vi "Pipelined Processing (Optimized Performance).vi"() -> ()   [LabVIEW 2023]
doc: "The Pipelined Processing (Optimized Performance) example shows how to use feedback nodes to allow different processing functions to operate on different images in the same cycle. This example uses a ring acquisition which is optimized for performance, but has some restrictions on the camera's image format and size. Use the Pipelined Processing VI if your camera settings do not work with a ring acquisition.\n\nIn this example, image processing is simulated by a time delay that can be adjusted while the VI is running. When processing is complete, <B>IMAQdx Release Image</B> must be called in order to free space in the ring buffer."
uses:
  <vilib>/vision/driver/IMAQdx.llb/IMAQdx Acquisition Mode.ctl
  <vilib>/vision/driver/IMAQdx.llb/IMAQdx Buffer Number Mode.ctl
  <vilib>/vision/Image Controls.llb/IMAQ Image.ctl
  <vilib>/vision/driver/NI_Vision_Acquisition_Software.lvlib
panel:
  in  "Processing Delay (ms)":dbl=5.0
  out "Image":T1(plugin-control)
  out "Acquired Frame Rate":dbl
  out "Processing Frame Rate":dbl
  in  "Enable Pipelined Processing":bool
  out "Lost Buffer Count":u32
  in  "Number of Images":i32=30
  in  "Camera Name":refnum<k21> caption="IMAQdx Session"
  in  "Stop":bool
  # "Overview: Demonstrates how to process an image using a pipelined approach to improve performance so multiple operations can happen on the same iteration of the loop.\nRequirements: Vision Acquisition Software\nInstructions:\n1. Select the Camera Name\n2. Run the VI and increase the Processing Delay until the Processing Frame Rate is less than the Acquired Frame Rate\n3. Stop the VI and turn on the Enabled Pipelined Processing and repeat step 2 to compare the maximum Processing Delay before falling behind"
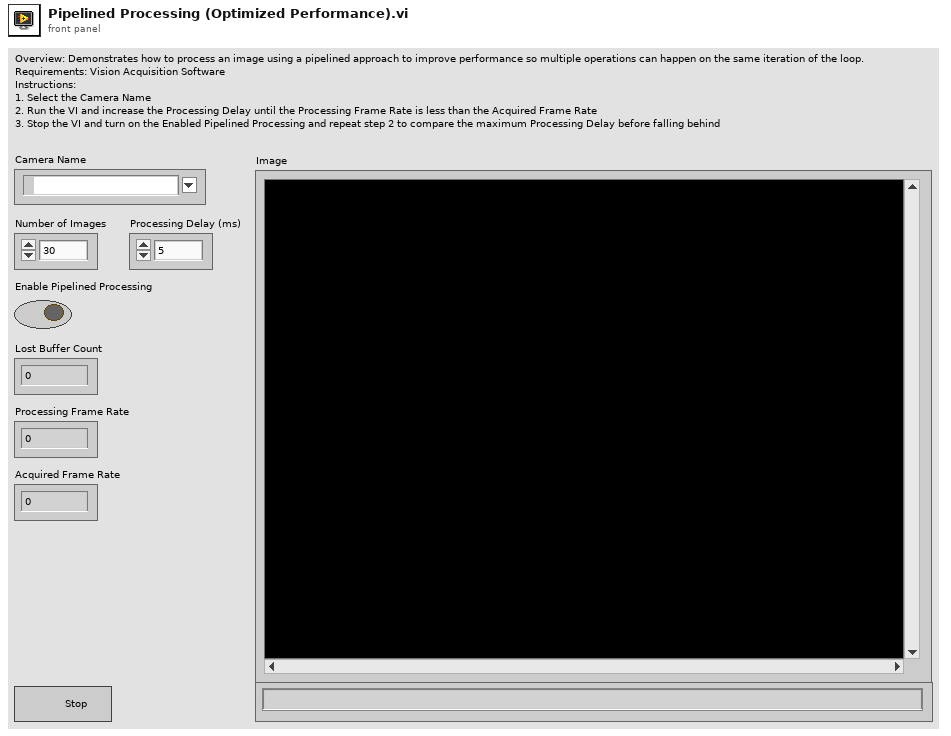
[diagram p1: front panel]
types:
  T1 = typedef "IMAQ Image.ctl" = refnum<image>
  T2 = typedef "NI_Vision_Acquisition_Software.lvlib/IMAQdx Acquisition Mode.ctl" = enum32{"One Shot", "Continuous"}
  T3 = typedef "IMAQdx.ctl" = refnum<k21>
  T4 = typedef "NI_Vision_Acquisition_Software.lvlib/IMAQdx Buffer Number Mode.ctl" = enum32{"Next", "Last", "Buffer Number", "Every", "Last New"}
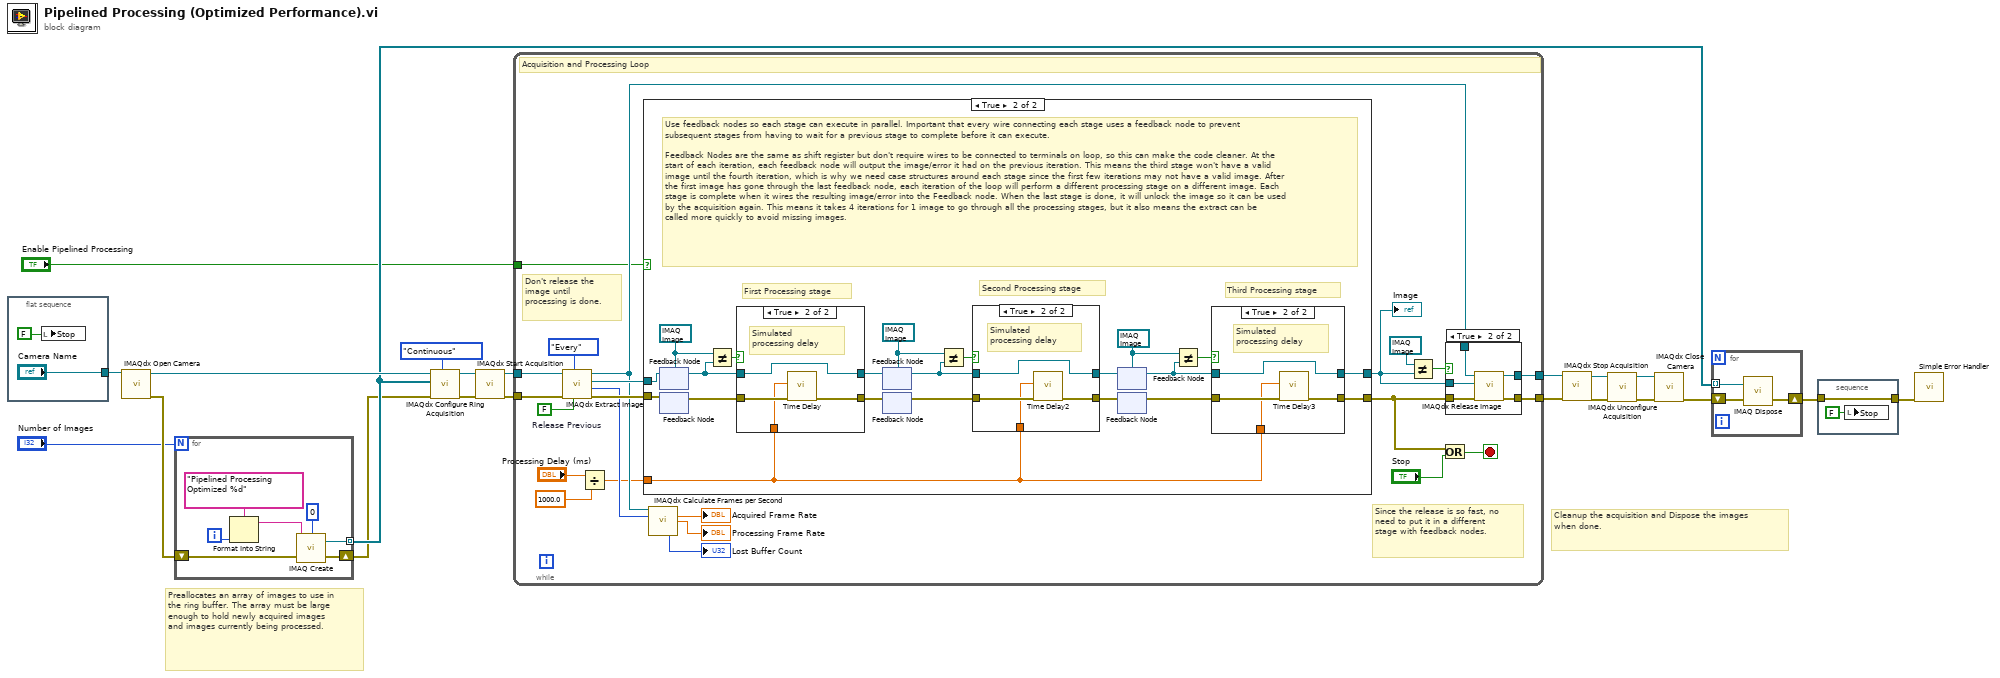
[diagram p0: block diagram]
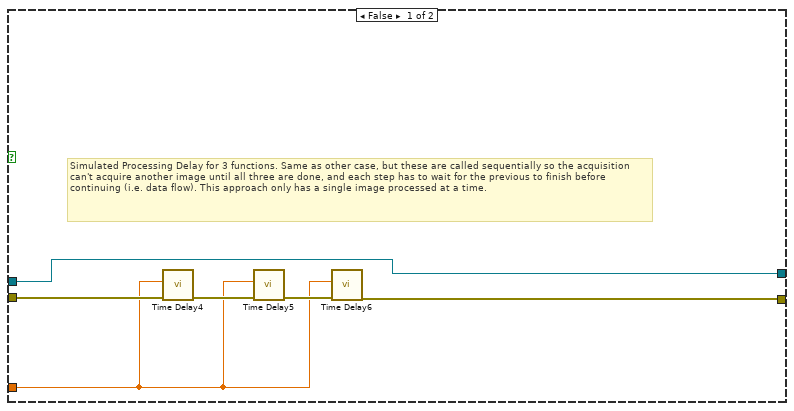
[diagram p2: hidden frame]
diagram:
  # "Cleanup the acquisition and Dispose the images when done."
  # "Preallocates an array of images to use in the ring buffer. The array must be large enough to hold newly acquired images and images currently being processed."
  n1 = flat-sequence {
    tunnel: ["Camera Name"] -> w20
    frame #0 {
      n2 = local write "Stop"(FALSE ("Stop")) -> ()
    }
  }
  n3 = call <vilib>:"IMAQdx Open Camera.vi"("Session In"=w20) -> ("error out"=w13:errorcluster, "Session Out"=w12:T3)  [unwired: 2 in, 7 out]
  n4 = for {
    N: "Number of Images" -> [_]
    tunnel: [w29] -> w9 mode=indexing
    shift-right: [w28] -> w4
    shift-left: w13 -> [w30]
    i -> [w27]
    n5 = Format Into String(format string="Pipelined Processing Optimized %d" ("Image Name"), w27) -> (resulting string=w26:string)  [unwired: 2 in, 1 out]
    n6 = call "IMAQ Create"("Border Size"=0, "Image Name"=w26, "error in (no error)"=w30) -> ("New Image"=w29:T1, "error out"=w28:errorcluster)  [unwired: 1 in, 1 out]
  }
  n7 = call <vilib>:"IMAQdx Configure Ring Acquisition.vi"("Mode"=IMAQdx_Acquisition_Mode."Continuous" ("Continuous?"), "error in"=w4, "Images"=w9, "Session In"=w12) -> ("error out"=w14:errorcluster, "Session Out"=w15:T3)  [unwired: 5 in, 1 out]
  n8 = call <vilib>:"IMAQdx Start Acquisition.vi"("error in"=w14, "Session In"=w15) -> ("error out"=w21:errorcluster, "Session Out"=w7:T3)  [unwired: 8 out]
  n9 = while {
    tunnel: w21 -> [w53]
    tunnel: w7 -> [w49]
    tunnel: [w41] -> w8
    tunnel: [w42] -> w1
    tunnel: "Enable Pipelined Processing" -> [w35]
    stop <- w36 stop-if-true
    w50 = FALSE  # Release Previous
    # "Since the release is so fast, no need to put it in a different stage with feedback nodes."
    # "Don't release the image until processing is done."
    # "Acquisition and Processing Loop"
    n10 = call <vilib>:"IMAQdx Extract Image.vi"("Release Previous (true)"=w50, "Buffer Number Mode (Next)"=IMAQdx_Buffer_Number_Mode."Every" ("Buffer Number Mode"), "error in"=w53, "Session In"=w49) -> ("error out"=w47:errorcluster, "Buffer Number Out"=w38:u32, "Image Out"=w46:T1, "Session Out"=w40:T3)  [unwired: 4 in]
    n11 = Divide(x="Processing Delay (ms)", y=1000.0) -> (x/y=w32:dbl)
    n12 = case shown="True" w35 {
      tunnel: w47 -> [w59 w80]
      tunnel: w46 -> [w55 w79]
      tunnel: [w56 w78] -> w43
      tunnel: [w55 w64] -> w31
      tunnel: w32 -> [w54 w60]
      frame False {
        # "Simulated Processing Delay for 3 functions. Same as other case, but these are called sequentially so the acquisition can't acquire another image until all three are done, and each step has to wait for the previous to finish before continuing (i.e. data flow). This approach only has a single image processed at a time."
        n13 = call "Time Delay4"("error in (no error)"=w59, "Delay Time (s)"=w54) -> ("error out"=w58:errorcluster)  [unwired: 9 in]
        n14 = call "Time Delay5"("error in (no error)"=w58, "Delay Time (s)"=w54) -> ("error out"=w57:errorcluster)  [unwired: 9 in]
        n15 = call "Time Delay6"("error in (no error)"=w57, "Delay Time (s)"=w54) -> ("error out"=w56:errorcluster)  [unwired: 9 in]
      }
      frame True {
        w61 = T1 refnum ("Image Out")
        w62 = T1 refnum ("Image Out")
        w63 = T1 refnum ("Image Out")
        # "Use feedback nodes so each stage can execute in parallel. Important that every wire connecting each stage uses a feedback node to prevent subsequent stages from having to wait for a previous stage to complete before it can execute.\n\nFeedback Nodes are the same as shift register but don't require wires to be connected to terminals on loop, so this can make the code cleaner. At the start of each iteration, each feedback node will output the image/error it had on the previous iteration. This means the third stage won't have a valid image until the fourth iteration, which is why we need case structures around each stage since the first few iterations may not have a valid image. After the first image has gone through the last feedback node, each iteration of the loop will perform a different processing stage on a different image. Each stage is complete when it wires the resulting image/error into the Feedback node. When the last stage is done, it will unlock the image so it can be used by the acquisition again. This means it takes 4 iterations for 1 image to go through all the processing stages, but it also means the extract can be called more quickly to avoid missing images."
        # "Third Processing stage"
        # "Second Processing stage"
        # "First Processing stage"
        n16 = feedback #1(w63) -> (w66:T1)
        n17 = feedback-in #1(w79) -> ()
        n18 = feedback #2() -> (w77:errorcluster)  [unwired: 1 in]
        n19 = feedback-in #2(w80) -> ()
        n20 = Not Equal?(x=w63, y=w66) -> (x != y?=w65:bool)
        n21 = case shown="True" w65 {
          tunnel: w77 -> [w93 w98]
          tunnel: w66 -> [w94 w95]
          tunnel: [w94 w95] -> w76
          tunnel: [w93 w97] -> w75
          tunnel: w60 -> [_ w96]
          frame False {
            # "No image to process"
          }
          frame True {
            # "Simulated processing delay"
            n22 = call "Time Delay"("error in (no error)"=w98, "Delay Time (s)"=w96) -> ("error out"=w97:errorcluster)  [unwired: 9 in]
          }
        }
        n23 = feedback #3(w62) -> (w73:T1)
        n24 = feedback-in #3(w76) -> ()
        n25 = feedback #4() -> (w72:errorcluster)  [unwired: 1 in]
        n26 = feedback-in #4(w75) -> ()
        n27 = Not Equal?(x=w62, y=w73) -> (x != y?=w74:bool)
        n28 = case shown="True" w74 {
          tunnel: w72 -> [w87 w92]
          tunnel: w73 -> [w88 w89]
          tunnel: [w88 w89] -> w71
          tunnel: [w87 w91] -> w70
          tunnel: w60 -> [_ w90]
          frame False {
            # "No image to process"
          }
          frame True {
            # "Simulated processing delay"
            n29 = call "Time Delay2"("error in (no error)"=w92, "Delay Time (s)"=w90) -> ("error out"=w91:errorcluster)  [unwired: 9 in]
          }
        }
        n30 = feedback #5(w61) -> (w69:T1)
        n31 = feedback-in #5(w71) -> ()
        n32 = feedback #6() -> (w68:errorcluster)  [unwired: 1 in]
        n33 = feedback-in #6(w70) -> ()
        n34 = Not Equal?(x=w61, y=w69) -> (x != y?=w67:bool)
        n35 = case shown="True" w67 {
          tunnel: w68 -> [w81 w86]
          tunnel: w69 -> [w82 w83]
          tunnel: [w82 w83] -> w64
          tunnel: [w81 w85] -> w78
          tunnel: w60 -> [_ w84]
          frame False {
            # "No image to process"
          }
          frame True {
            # "Simulated processing delay"
            n36 = call "Time Delay3"("error in (no error)"=w86, "Delay Time (s)"=w84) -> ("error out"=w85:errorcluster)  [unwired: 9 in]
          }
        }
      }
    }
    "Image" <- w31
    n37 = call <vilib>:"IMAQdx Calculate Frames per Second.vi"("Session In"=w40, "Buffer Number"=w38) -> ("Acquired Frames per Second"=→"Acquired Frame Rate":dbl, "Processed Frames per Second"=→"Processing Frame Rate":dbl, "Images Missed"=→"Lost Buffer Count":u32)  [unwired: 7 in, 4 out]
    n38 = Not Equal?(x=T1 refnum ("Image Out"), y=w31) -> (x != y?=w39:bool)
    n39 = Or(x=w43, y="Stop") -> (x .or. y?=w36:bool)
    n40 = case shown="True" w39 {
      tunnel: w43 -> [w100 w105]
      tunnel: [w100 w104] -> w42
      tunnel: [w99 w103] -> w41
      tunnel: w40 -> [w99 w102]
      tunnel: w31 -> [_ w101]
      frame False {
      }
      frame True {
        n41 = call <vilib>:"IMAQdx Release Image.vi"("error in"=w105, "Image"=w101, "Session In"=w102) -> ("error out"=w104:errorcluster, "Session Out"=w103:T3)  [unwired: 7 in]
      }
    }
  }
  n42 = call <vilib>:"IMAQdx Stop Acquisition.vi"("error in"=w1, "Session In"=w8) -> ("error out"=w16:errorcluster, "Session Out"=w17:T3)  [unwired: 8 out]
  n43 = call <vilib>:"IMAQdx Unconfigure Acquisition.vi"("error in"=w16, "Session In"=w17) -> ("error out"=w19:errorcluster, "Session Out"=w18:T3)  [unwired: 8 out]
  n44 = call <vilib>:"IMAQdx Close Camera.vi"("error in"=w19, "Session In"=w18) -> ("error out"=w3:errorcluster)  [unwired: 9 out]
  n45 = for {
    shift-right: [w107] -> w6
    shift-left: w3 -> [w108]
    tunnel: w9 -> [w106] mode=indexing
    n46 = call "IMAQ Dispose"("Image"=w106, "error in (no error)"=w108) -> ("error out"=w107:errorcluster)  [unwired: 4 in]
  }
  n47 = stacked-sequence {
    tunnel: [w109] -> w5
    tunnel: w6 -> [w109]
    frame #0 {
      n48 = local write "Stop"(FALSE ("Stop")) -> ()
    }
  }
  n49 = call <vilib>:"Simple Error Handler.vi"("error in (no error)"=w5) -> ()  [unwired: 4 in, 5 out]
